vi "FPServer.vi"   [LabVIEW 2014]
uses:
  WebFrontPanel_class/WebFrontPanel.lvclass
  FrontPanelManager_class/FrontPanelManager.lvclass
types:
  T1 = typedef "Message.ctl" = cluster{"Message":string, "Data":variant, "Response":refnum<queue>}
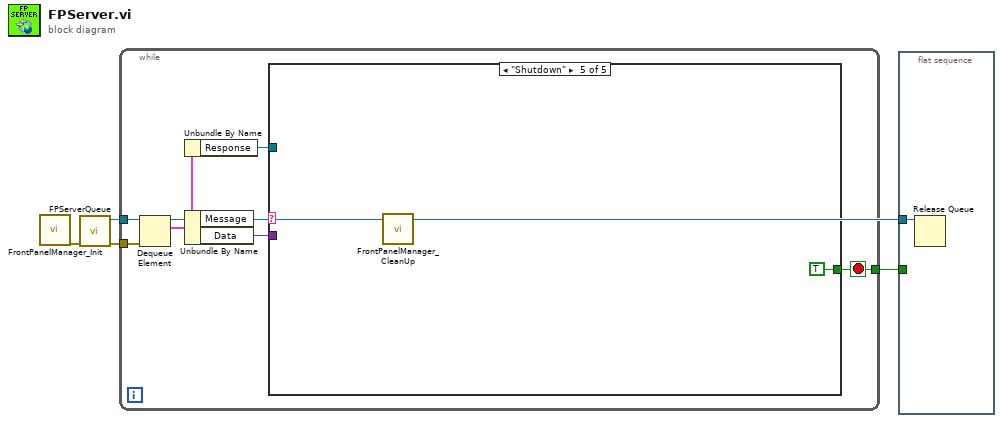
[diagram p0: block diagram]
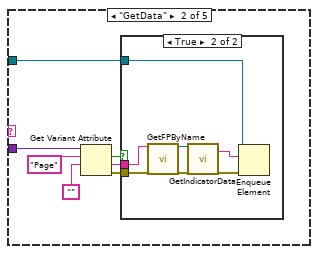
[diagram p3: hidden frame]
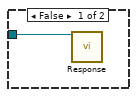
[diagram p4: hidden frame]
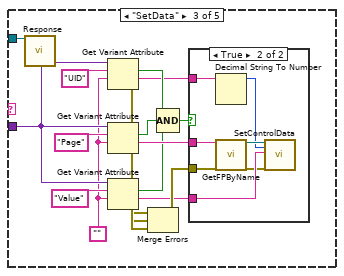
[diagram p5: hidden frame]
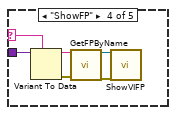
[diagram p7: hidden frame]
diagram:
  n1 = call "FrontPanelManager_Init.vi"() -> ("error out"=w2:errorcluster)  [unwired: 18 in, 1 out]
  n2 = call "FPServerQueue.vi"("error in (no error)"=w2) -> ("FPServer Queue"=w3:refnum<queue>, "error out"=w1:errorcluster)  [unwired: 9 in]
  n3 = while {
    tunnel: w3 -> [w11]
    tunnel: [w6] -> w4
    tunnel: w1 -> [w5]
    stop <- w6 stop-if-true
    n4 = Dequeue Element(queue=w11, error in (no error)=w5) -> (element=w8:T1)  [unwired: 1 in, 3 out]
    n5 = Unbundle By Name(w8) -> ("Response"=w7:refnum<queue>)
    n6 = Unbundle By Name(w8) -> ("Message"=w10:string, "Data"=w9:variant)
    n7 = case shown="\"Shutdown\"" w10 {
      selector: w10 -> [_ _ _ w55 _]
      tunnel: w9 -> [_ w17 w36 w56 _]
      tunnel: [_ _ _ _ TRUE] -> w6
      tunnel: w7 -> [_ w18 w43 _ _]
      frame Default {
      }
      frame "GetData" {
        n8 = Get Variant Attribute(Variant=w17, name="Page", default value (empty Variant)="") -> (found=w14:bool, value=w12:string, error out=w15:errorcluster)  [unwired: 1 in, 1 out]
        n9 = case shown="True" w14 {
          tunnel: w18 -> [w19 w24]
          tunnel: w15 -> [_ w21]
          tunnel: w12 -> [_ w20]
          frame False {
            n10 = call "Response.vi"("Response"=w19) -> ()  [unwired: 19 in]
          }
          frame True {
            n11 = call "GetFPByName.vi"("WFP Name"=w20, "error in (no error)"=w21) -> ("WebFrontPanel"=w26:refnum<class "WebFrontPanel.lvclass">, "error out"=w25:errorcluster)  [unwired: 15 in, 1 out]
            n12 = call-dynamic "GetIndicatorData.vi"("reference in"=w26, "error in (no error)"=w25) -> ("String"=w23:string, "error out"=w22:errorcluster)  [unwired: 15 in, 1 out]
            n13 = Enqueue Element(queue=w24, element=w23, error in (no error)=w22) -> ()  [unwired: 1 in, 3 out]
          }
        }
      }
      frame "SetData" {
        w27 = ""
        n14 = call "Response.vi"("Response"=w43) -> ()  [unwired: 19 in]
        n15 = Get Variant Attribute(Variant=w36, name="UID", default value (empty Variant)=w27) -> (found=w35:bool, value=w33:string, error out=w31:errorcluster)  [unwired: 1 in, 1 out]
        n16 = Get Variant Attribute(Variant=w36, name="Page", default value (empty Variant)=w27) -> (found=w34:bool, value=w40:string, error out=w32:errorcluster)  [unwired: 1 in, 1 out]
        n17 = Get Variant Attribute(Variant=w36, name="Value", default value (empty Variant)=w27) -> (found=w37:bool, value=w28:string, error out=w30:errorcluster)  [unwired: 1 in, 1 out]
        n18 = Merge Errors(w30, w31, w32) -> (w29:errorcluster)
        n19 = Compound Arithmetic op=AND(w35, w34, w37) -> (w39:bool)
        n20 = case shown="True" w39 {
          tunnel: w40 -> [_ w50]
          tunnel: w29 -> [_ w49]
          tunnel: w33 -> [_ w47]
          tunnel: w28 -> [_ w45]
          frame False {
          }
          frame True {
            n21 = Decimal String To Number(string=w47) -> (number=w46:i32)  [unwired: 2 in, 1 out]
            n22 = call "GetFPByName.vi"("WFP Name"=w50, "error in (no error)"=w49) -> ("WebFrontPanel"=w48:refnum<class "WebFrontPanel.lvclass">, "error out"=w44:errorcluster)  [unwired: 15 in, 1 out]
            n23 = call-dynamic "SetControlData.vi"("reference in"=w48, "UID"=w46, "Value"=w45, "error in (no error)"=w44) -> ()  [unwired: 14 in, 2 out]
          }
        }
      }
      frame "ShowFP" {
        n24 = Variant To Data(type=w55, Variant=w56) -> (data=w54:string, error out=w53:errorcluster)  [unwired: 1 in]
        n25 = call "GetFPByName.vi"("WFP Name"=w54, "error in (no error)"=w53) -> ("WebFrontPanel"=w52:refnum<class "WebFrontPanel.lvclass">, "error out"=w51:errorcluster)  [unwired: 15 in, 1 out]
        n26 = call-dynamic "ShowVIFP.vi"("reference in"=w52, "error in (no error)"=w51) -> ()  [unwired: 16 in, 2 out]
      }
      frame "Shutdown" {
        n27 = call "FrontPanelManager_CleanUp.vi"() -> ()  [unwired: 19 in, 1 out]
      }
    }
  }
  n28 = flat-sequence {
    tunnel: w3 -> [w58]
    tunnel: w4 -> [_]
    frame #0 {
      n29 = Release Queue(queue=w58) -> ()  [unwired: 2 in, 3 out]
    }
  }
